vi "Required And Outputs.vi"(0 "Numeric":dbl=1122.0, 5 "Cluster":cluster{"String":string, "Time Stamp":timestamp}={"String"="aaaa", "Time Stamp"=timestamp(3383145346.3459997 s since 1904-01-01)}, 9 "Array":T2(array[cluster])=[{"String"="aaaaabbbb", "Time Stamp"=timestamp(3383663965.7679996 s since 1904-01-01)}]) -> (3 "Cluster 2":cluster{"String":string, "Numeric 2":dbl}={"String"="output", "Numeric 2"=4455.0}, 4 "String":string="output", 6 "Numeric 2":dbl=4455.0, 8 "Enum":enum16{"aaaa", "bbbb", "cccc"}(ring)=enum."cccc", 10 "Boolean":bool=TRUE, 14 "Array 2":T1(array[cluster])=[{"String"="Should not show this value", "Numeric 2"=7788.0, "Enum"=enum."bbbb"}], 15 "error out":errorcluster)   [LabVIEW 2011]
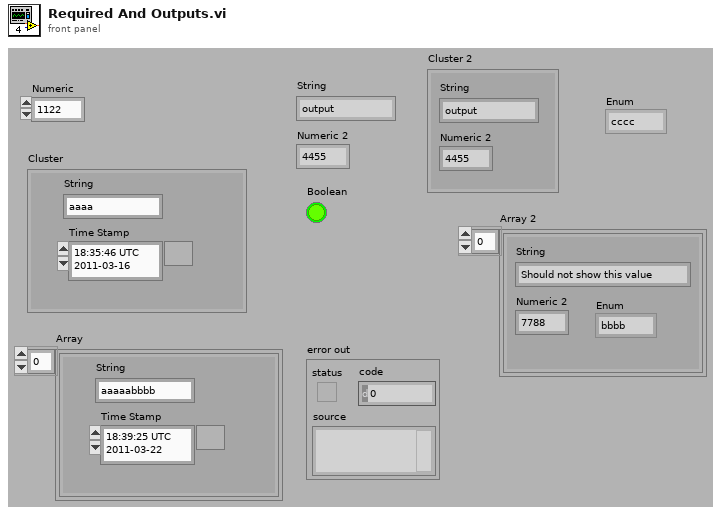
[diagram p1: front panel]
types:
  T1 = cluster{"String":string, "Numeric 2":dbl, "Enum":enum16{"aaaa", "bbbb", "cccc"}}[]
  T2 = cluster{"String":string, "Time Stamp":timestamp}[]
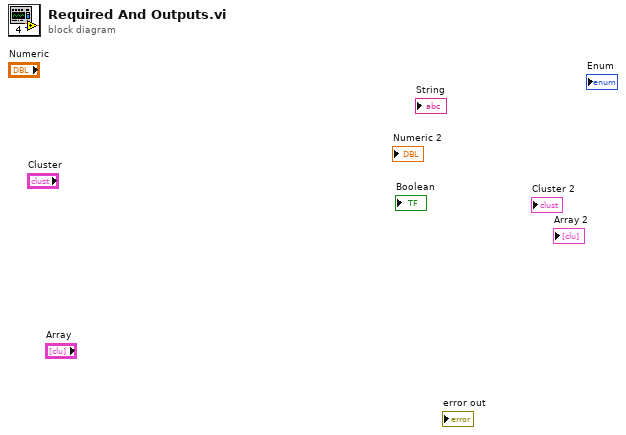
[diagram p0: block diagram]
diagram:
